vi "Login_dialog.vi"() -> (2 "Experiment title out":string, 3 "User name out":string)   [LabVIEW 2016]
panel:
  in  "Login":bool
  in  "Experiment title":string
  in  "User name":string
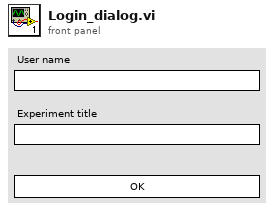
[diagram p1: front panel]
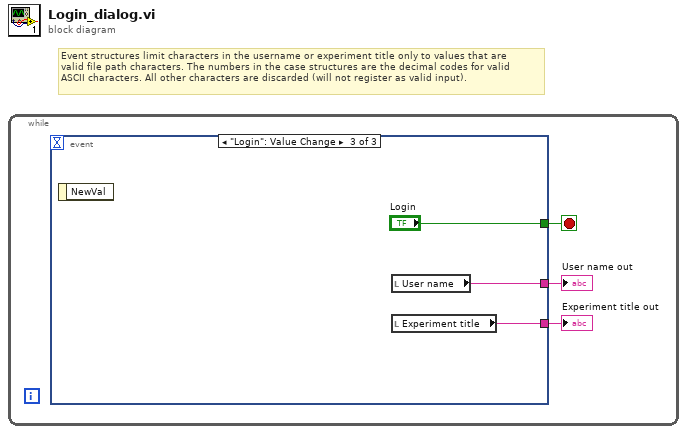
[diagram p0: block diagram]
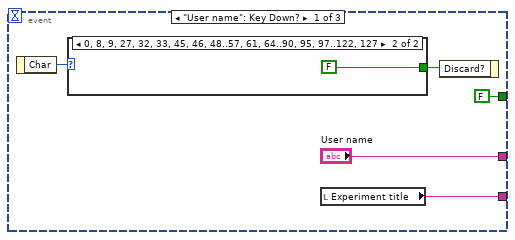
[diagram p2: hidden frame]
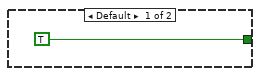
[diagram p3: hidden frame]
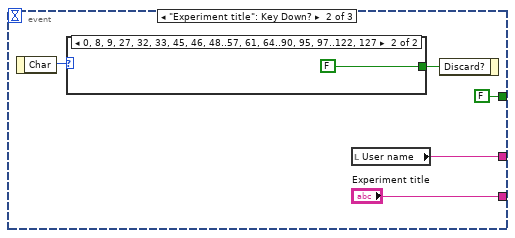
[diagram p4: hidden frame]
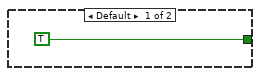
[diagram p5: hidden frame]
diagram:
  # "Event structures limit characters in the username or experiment title only to values that are\nvalid file path characters. The numbers in the case structures are the decimal codes for valid\nASCII characters. All other characters are discarded (will not register as valid input)."
  n1 = while {
    stop <- w3 stop-if-true
    n2 = event shown="[2] \"Login\": Value Change" {
      selector: _ -> [_ _ _]
      dyn-events: _ -> [_ _ _]
      timeout: _ -> [_ _ _]
      tunnel: [FALSE ("NewVal") FALSE ("NewVal") "Login"] -> w3
      tunnel: ["User name" w12 w19] -> w2
      tunnel: [w4 "Experiment title" w18] -> w1
      event "User name": Key Down? {
        n3 = event-data() -> ("Char"=w8:i16)  [unwired: 1 in]
        n4 = case shown="0, 8, 9, 27, 32, 33, 45, 46, 48..57, 61, 64..90, 95, 97..122, 127" w8 {
          tunnel: [TRUE FALSE] -> w7
          frame Default {
          }
          frame 0, 8, 9, 27, 32, 33, 45, 46, 48..57, 61, 64..90, 95, 97..122, 127 {
          }
        }
        n5 = local read "Experiment title"() -> (w4:string)
        n6 = event-data("Discard?"=w7) -> ()  [unwired: 1 in, 1 out]
      }
      event "Experiment title": Key Down? {
        n7 = event-data() -> ("Char"=w15:i16)  [unwired: 1 in]
        n8 = case shown="0, 8, 9, 27, 32, 33, 45, 46, 48..57, 61, 64..90, 95, 97..122, 127" w15 {
          tunnel: [TRUE FALSE] -> w14
          frame Default {
          }
          frame 0, 8, 9, 27, 32, 33, 45, 46, 48..57, 61, 64..90, 95, 97..122, 127 {
          }
        }
        n9 = local read "User name"() -> (w12:string)
        n10 = event-data("Discard?"=w14) -> ()  [unwired: 1 in, 1 out]
      }
      event "Login": Value Change {
        n11 = event-data() -> ()  [unwired: 1 in, 1 out]
        n12 = local read "User name"() -> (w19:string)
        n13 = local read "Experiment title"() -> (w18:string)
      }
    }
    "User name out" <- w2
    "Experiment title out" <- w1
  }
